vi "IVA_Actividad_04.vi"() -> ()   [LabVIEW 2025]
uses:
  <vilib>/DAQmx/read.llb/DAQmx Read (Digital 1D Bool 1Chan 1Samp).vi
  <vilib>/DAQmx/create/channels.llb/DAQmx Create Channel (DI-Digital Input).vi
  <vilib>/DAQmx/miscellaneous.llb/DAQmx Fill In Error Info.vi
panel:
  out "A 2":bool
  in  "stop":bool
  out "B":bool
  out "A":bool
  out "Count":dbl
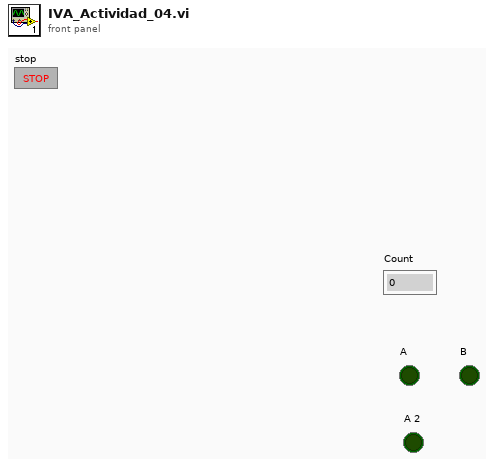
[diagram p1: front panel]
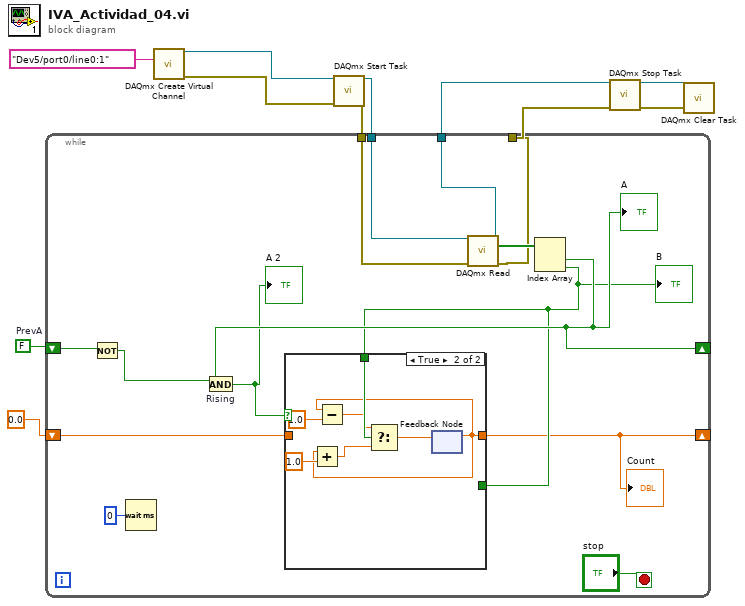
[diagram p0: block diagram]
diagram:
  w11 = FALSE  # PrevA
  n1 = call-poly <vilib>:"DAQmx Create Virtual Channel.vi"("lines"=tag "Dev5/port0/line0:1") -> ("task out"=w4:refnum<k21>, "error out"=w3:errorcluster)  [unwired: 13 in]
  n2 = call <vilib>:"DAQmx Start Task.vi"("task/channels in"=w4, "error in"=w3) -> ("task out"=w2:refnum<k21>, "error out"=w1:errorcluster)  [unwired: 12 in]
  n3 = while {
    shift-right: [w20] -> _
    shift-left: w11 -> [w23]
    shift-right: [w13] -> _
    shift-left: 0.0 ("Count") -> [w21]
    tunnel: [w19] -> w9
    tunnel: [w18] -> w7
    tunnel: w2 -> [w15]
    tunnel: w1 -> [w14]
    stop <- "stop" stop-if-true
    n4 = Not(x=w23) -> (.not. x?=w22:bool)
    n5 = Wait (ms)(milliseconds to wait=u32 0) -> ()  [unwired: 1 out]
    n6 = call-poly <vilib>:"DAQmx Read.vi"("task/channels in"=w15, "error in"=w14) -> ("task out"=w18:refnum<k21>, "data"=w24:bool[], "error out"=w19:errorcluster)  [unwired: 11 in]
    n7 = Index Array(array=w24) -> (element #1=w20:bool, element #2=w16:bool)  [unwired: 2 in]
    "A" <- w20
    "B" <- w16
    n8 = And "Rising"(x=w22, y=w20) -> (x .and. y?=w12:bool)
    "A 2" <- w12
    n9 = case shown="True" w12 {
      tunnel: w21 -> [w26 _]
      tunnel: w16 -> [_ _]
      tunnel: [w26 w27] -> w13
      tunnel: w16 -> [_ w33]
      frame False {
      }
      frame True {
        n10 = feedback #1() -> (w27:dbl)  [unwired: 1 in]
        n11 = Add(x=w27, y=1.0) -> (x+y=w31:dbl)
        n12 = Subtract(x=w27, y=1.0) -> (x-y=w29:dbl)
        n13 = Select(t=w29, s=w33, f=w31) -> (s? t:f=w28:dbl)
        n14 = feedback-in #1(w28) -> ()
      }
    }
    "Count" <- w13
  }
  n15 = call <vilib>:"DAQmx Stop Task.vi"("task/channels in"=w7, "error in"=w9) -> ("task out"=w6:refnum<k21>, "error out"=w8:errorcluster)  [unwired: 12 in]
  n16 = call <vilib>:"DAQmx Clear Task.vi"("task in"=w6, "error in"=w8) -> ()  [unwired: 13 in, 1 out]
